vi "Day 5 (Part One).vi"() -> ()   [LabVIEW 2021]
panel:
  out "Result":string
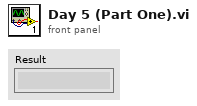
[diagram p1: front panel]
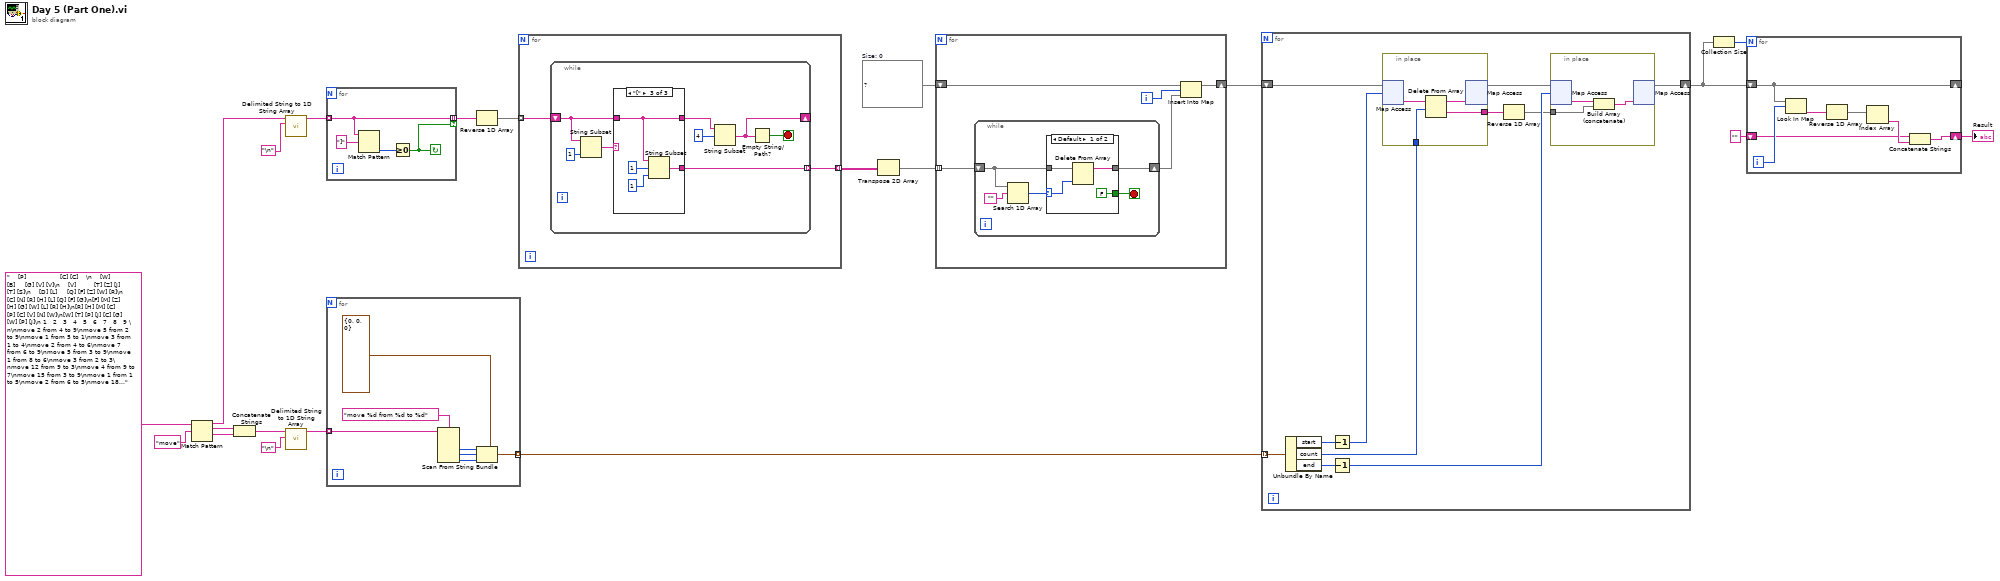
[diagram p0: block diagram]
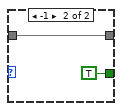
[diagram p2: hidden frame]
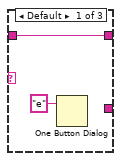
[diagram p3: hidden frame]
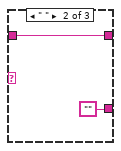
[diagram p4: hidden frame]
diagram:
  w7 = map{i32, string[]} {}  # Size: 0
  n1 = Match Pattern(string="    [P]                 [C] [C]    \n    [W]         [B]     [G] [V] [V]\n    [V]         [T] [Z] [J] [T] [S]\n    [D] [L]     [Q] [F] [Z] [W] [R]\n    [C] [N] [R] [H] [L] [Q] [F] [G]\n[F] [M] [Z] [H] [G] [W] [L] [R] [H]\n[R] [H] [M] [C] [P] [C] [V] [N] [W]\n[W] [T] [P] [J] [C] [G] [W] [P] [J]\n 1   2   3   4   5   6   7   8   9 \n\nmove 2 from 4 to 9\nmove 5 from 2 to 9\nmove 1 from 5 to 1\nmove 3 from 1 to 4\nmove 2 from 4 to 6\nmove 7 from 6 to 9\nmove 5 from 3 to 9\nmove 1 from 8 to 6\nmove 3 from 2 to 3\nmove 12 from 9 to 3\nmove 4 from 9 to 7\nmove 15 from 3 to 9\nmove 1 from 1 to 5\nmove 2 from 6 to 5\nmove 18 from 9 to 1\nmove 6 from 8 to 1\nmove 1 from 8 to 7\nmove 5 from 7 to 2\nmove 6 from 1 to 2\nmove 7 from 9 to 6\nmove 6 from 1 to 3\nmove 5 from 3 to 9\nmove 3 from 9 to 1\nmove 1 from 7 to 9\nmove 4 from 2 to 1\nmove 5 from 6 to 3\nmove 1 from 3 to 4\nmove 1 from 5 to 9\nmove 2 from 9 to 6\nmove 5 from 5 to 9\nmove 10 from 1 to 8\nmove 4 from 3 to 8\nmove 3 from 4 to 9\nmove 4 from 6 to 9\nmove 14 from 8 to 6\nmove 1 from 3 to 8\nmove 14 from 9 to 4\nmove 6 from 1 to 6\nmove 1 from 8 to 2\nmove 3 from 5 to 8\nmove 1 from 8 to 9\nmove 1 from 8 to 1\nmove 5 from 4 to 9\nmove 1 from 8 to 4\nmove 3 from 9 to 4\nmove 3 from 7 to 5\nmove 7 from 6 to 3\nmove 7 from 4 to 1\nmove 3 from 9 to 1\nmove 7 from 2 to 3\nmove 1 from 4 to 8\nmove 8 from 6 to 2\nmove 2 from 7 to 4\nmove 1 from 7 to 4\nmove 1 from 7 to 9\nmove 1 from 5 to 9\nmove 1 from 9 to 4\nmove 1 from 4 to 2\nmove 8 from 4 to 9\nmove 1 from 4 to 2\nmove 5 from 9 to 4\nmove 2 from 6 to 9\nmove 1 from 6 to 9\nmove 1 from 8 to 1\nmove 13 from 3 to 2\nmove 1 from 3 to 9\nmove 2 from 6 to 8\nmove 1 from 8 to 1\nmove 14 from 1 to 7\nmove 4 from 2 to 1\nmove 2 from 9 to 5\nmove 3 from 9 to 7\nmove 1 from 8 to 2\nmove 4 from 1 to 5\nmove 1 from 4 to 7\nmove 3 from 9 to 1\nmove 7 from 7 to 4\nmove 14 from 2 to 8\nmove 3 from 1 to 7\nmove 3 from 5 to 4\nmove 2 from 1 to 9\nmove 11 from 8 to 9\nmove 3 from 7 to 8\nmove 3 from 8 to 6\nmove 6 from 4 to 3\nmove 2 from 6 to 8\nmove 8 from 4 to 3\nmove 3 from 8 to 7\nmove 2 from 8 to 2\nmove 2 from 3 to 9\nmove 1 from 6 to 8\nmove 5 from 2 to 7\nmove 10 from 9 to 7\nmove 1 from 8 to 5\nmove 3 from 5 to 2\nmove 6 from 7 to 5\nmove 19 from 7 to 3\nmove 9 from 5 to 9\nmove 6 from 2 to 6\nmove 2 from 7 to 3\nmove 29 from 3 to 8\nmove 2 from 7 to 9\nmove 5 from 8 to 1\nmove 12 from 9 to 6\nmove 1 from 3 to 8\nmove 1 from 2 to 7\nmove 1 from 3 to 1\nmove 10 from 6 to 1\nmove 1 from 6 to 7\nmove 9 from 1 to 9\nmove 2 from 1 to 2\nmove 12 from 9 to 4\nmove 7 from 6 to 3\nmove 8 from 3 to 7\nmove 5 from 7 to 6\nmove 19 from 8 to 3\nmove 10 from 4 to 6\nmove 1 from 4 to 6\nmove 6 from 8 to 6\nmove 1 from 4 to 2\nmove 6 from 6 to 3\nmove 3 from 2 to 7\nmove 13 from 6 to 3\nmove 1 from 9 to 1\nmove 6 from 1 to 8\nmove 1 from 6 to 5\nmove 1 from 5 to 4\nmove 3 from 7 to 1\nmove 2 from 1 to 3\nmove 11 from 3 to 8\nmove 1 from 4 to 3\nmove 3 from 8 to 4\nmove 1 from 7 to 5\nmove 3 from 8 to 9\nmove 2 from 9 to 2\nmove 7 from 8 to 3\nmove 1 from 7 to 9\nmove 1 from 1 to 4\nmove 32 from 3 to 4\nmove 1 from 5 to 9\nmove 2 from 8 to 3\nmove 2 from 6 to 4\nmove 1 from 9 to 4\nmove 1 from 9 to 2\nmove 3 from 3 to 1\nmove 1 from 8 to 6\nmove 1 from 6 to 2\nmove 1 from 9 to 3\nmove 1 from 1 to 7\nmove 1 from 8 to 7\nmove 2 from 3 to 8\nmove 1 from 8 to 4\nmove 1 from 1 to 2\nmove 2 from 4 to 8\nmove 1 from 1 to 8\nmove 26 from 4 to 6\nmove 3 from 8 to 5\nmove 3 from 7 to 6\nmove 7 from 6 to 3\nmove 18 from 6 to 8\nmove 16 from 8 to 9\nmove 1 from 5 to 1\nmove 2 from 8 to 3\nmove 3 from 9 to 8\nmove 3 from 6 to 4\nmove 2 from 5 to 4\nmove 1 from 6 to 4\nmove 2 from 7 to 2\nmove 2 from 3 to 9\nmove 4 from 8 to 3\nmove 1 from 1 to 2\nmove 6 from 9 to 7\nmove 2 from 2 to 5\nmove 12 from 3 to 1\nmove 9 from 9 to 2\nmove 10 from 1 to 3\nmove 2 from 5 to 9\nmove 8 from 4 to 7\nmove 13 from 7 to 6\nmove 6 from 6 to 5\nmove 4 from 5 to 3\nmove 2 from 5 to 4\nmove 8 from 4 to 3\nmove 1 from 7 to 2\nmove 15 from 2 to 7\nmove 8 from 3 to 7\nmove 1 from 1 to 6\nmove 7 from 7 to 1\nmove 5 from 1 to 6\nmove 7 from 3 to 2\nmove 3 from 1 to 6\nmove 12 from 7 to 9\nmove 12 from 9 to 8\nmove 1 from 7 to 1\nmove 2 from 9 to 5\nmove 1 from 1 to 9\nmove 4 from 4 to 2\nmove 4 from 8 to 4\nmove 2 from 7 to 2\nmove 4 from 6 to 5\nmove 4 from 8 to 9\nmove 1 from 8 to 4\nmove 5 from 5 to 3\nmove 5 from 2 to 4\nmove 5 from 9 to 5\nmove 1 from 3 to 6\nmove 1 from 7 to 8\nmove 12 from 3 to 9\nmove 4 from 2 to 6\nmove 7 from 4 to 9\nmove 13 from 6 to 4\nmove 3 from 6 to 9\nmove 4 from 4 to 2\nmove 1 from 3 to 4\nmove 21 from 9 to 7\nmove 4 from 2 to 1\nmove 3 from 5 to 4\nmove 8 from 7 to 6\nmove 2 from 7 to 2\nmove 11 from 4 to 2\nmove 1 from 9 to 7\nmove 1 from 5 to 7\nmove 1 from 1 to 8\nmove 5 from 2 to 5\nmove 1 from 3 to 5\nmove 2 from 4 to 9\nmove 3 from 4 to 8\nmove 3 from 1 to 8\nmove 1 from 9 to 6\nmove 8 from 7 to 8\nmove 9 from 6 to 5\nmove 1 from 9 to 6\nmove 1 from 6 to 4\nmove 3 from 7 to 5\nmove 1 from 6 to 9\nmove 12 from 5 to 1\nmove 2 from 5 to 8\nmove 1 from 9 to 6\nmove 2 from 7 to 6\nmove 9 from 1 to 8\nmove 1 from 6 to 9\nmove 1 from 9 to 2\nmove 1 from 4 to 2\nmove 2 from 6 to 7\nmove 5 from 8 to 3\nmove 2 from 7 to 4\nmove 16 from 8 to 5\nmove 2 from 3 to 8\nmove 7 from 5 to 1\nmove 3 from 3 to 8\nmove 7 from 5 to 7\nmove 4 from 5 to 2\nmove 6 from 7 to 9\nmove 2 from 9 to 6\nmove 2 from 9 to 2\nmove 1 from 6 to 8\nmove 12 from 2 to 6\nmove 2 from 9 to 6\nmove 1 from 5 to 2\nmove 3 from 5 to 4\nmove 9 from 2 to 6\nmove 6 from 8 to 3\nmove 1 from 7 to 5\nmove 1 from 6 to 7\nmove 1 from 7 to 8\nmove 1 from 5 to 8\nmove 5 from 1 to 2\nmove 3 from 4 to 5\nmove 4 from 6 to 8\nmove 5 from 2 to 9\nmove 5 from 8 to 4\nmove 1 from 1 to 4\nmove 9 from 8 to 4\nmove 1 from 2 to 3\nmove 3 from 6 to 8\nmove 4 from 9 to 2\nmove 2 from 6 to 4\nmove 2 from 3 to 1\nmove 4 from 4 to 7\nmove 6 from 4 to 5\nmove 10 from 6 to 8\nmove 4 from 1 to 9\nmove 4 from 7 to 5\nmove 3 from 3 to 9\nmove 6 from 9 to 8\nmove 2 from 2 to 9\nmove 8 from 4 to 3\nmove 2 from 2 to 7\nmove 1 from 4 to 9\nmove 6 from 3 to 8\nmove 2 from 7 to 8\nmove 6 from 5 to 9\nmove 5 from 5 to 6\nmove 2 from 5 to 9\nmove 7 from 9 to 5\nmove 2 from 1 to 9\nmove 6 from 5 to 8\nmove 1 from 5 to 1\nmove 2 from 3 to 6\nmove 1 from 3 to 6\nmove 4 from 9 to 5\nmove 1 from 3 to 4\nmove 1 from 1 to 2\nmove 1 from 2 to 1\nmove 1 from 6 to 8\nmove 14 from 8 to 5\nmove 6 from 5 to 1\nmove 16 from 8 to 3\nmove 2 from 8 to 2\nmove 10 from 6 to 7\nmove 1 from 6 to 9\nmove 2 from 2 to 9\nmove 2 from 7 to 3\nmove 1 from 8 to 5\nmove 3 from 9 to 1\nmove 4 from 9 to 5\nmove 9 from 3 to 8\nmove 2 from 3 to 6\nmove 5 from 3 to 8\nmove 1 from 4 to 2\nmove 12 from 8 to 4\nmove 1 from 8 to 9\nmove 4 from 5 to 9\nmove 7 from 7 to 1\nmove 10 from 5 to 2\nmove 2 from 5 to 2\nmove 1 from 6 to 5\nmove 2 from 5 to 2\nmove 5 from 2 to 6\nmove 4 from 9 to 6\nmove 6 from 4 to 9\nmove 2 from 3 to 4\nmove 6 from 4 to 7\nmove 6 from 7 to 5\nmove 10 from 1 to 5\nmove 4 from 1 to 2\nmove 4 from 6 to 3\nmove 6 from 9 to 7\nmove 2 from 4 to 9\nmove 7 from 7 to 6\nmove 1 from 9 to 7\nmove 2 from 9 to 8\nmove 2 from 8 to 2\nmove 1 from 2 to 5\nmove 3 from 8 to 4\nmove 4 from 2 to 7\nmove 3 from 4 to 7\nmove 2 from 3 to 5\nmove 2 from 3 to 2\nmove 18 from 5 to 3\nmove 6 from 3 to 1\nmove 8 from 3 to 1\nmove 8 from 7 to 9\nmove 9 from 2 to 5\nmove 3 from 2 to 3\nmove 7 from 3 to 7\nmove 3 from 6 to 4\nmove 1 from 7 to 1\nmove 7 from 6 to 7\nmove 1 from 2 to 9\nmove 1 from 4 to 2\nmove 13 from 7 to 2\nmove 10 from 5 to 3\nmove 1 from 2 to 9\nmove 7 from 1 to 5\nmove 8 from 9 to 5\nmove 1 from 9 to 5\nmove 1 from 9 to 8\nmove 1 from 8 to 2\nmove 8 from 5 to 3\nmove 18 from 3 to 5\nmove 2 from 4 to 1\nmove 3 from 2 to 5\nmove 27 from 5 to 1\nmove 17 from 1 to 5\nmove 2 from 2 to 3\nmove 1 from 6 to 5\nmove 2 from 2 to 5\nmove 1 from 6 to 4\nmove 1 from 6 to 9\nmove 2 from 3 to 5\nmove 17 from 5 to 6\nmove 1 from 9 to 3\nmove 6 from 2 to 4\nmove 1 from 3 to 2\nmove 3 from 4 to 9\nmove 1 from 2 to 9\nmove 1 from 4 to 7\nmove 3 from 5 to 2\nmove 2 from 5 to 1\nmove 1 from 5 to 2\nmove 1 from 7 to 3\nmove 18 from 1 to 4\nmove 1 from 3 to 1\nmove 5 from 4 to 2\nmove 1 from 5 to 1\nmove 9 from 2 to 7\nmove 1 from 4 to 5\nmove 1 from 2 to 9\nmove 8 from 6 to 2\nmove 13 from 4 to 2\nmove 2 from 4 to 9\nmove 1 from 5 to 2\nmove 1 from 6 to 8\nmove 6 from 7 to 5\nmove 1 from 8 to 4\nmove 1 from 7 to 6\nmove 1 from 6 to 1\nmove 7 from 6 to 5\nmove 1 from 7 to 9\nmove 6 from 9 to 3\nmove 2 from 9 to 7\nmove 2 from 5 to 7\nmove 4 from 7 to 8\nmove 4 from 5 to 4\nmove 1 from 6 to 7\nmove 3 from 3 to 8\nmove 6 from 5 to 9\nmove 2 from 3 to 5\nmove 4 from 4 to 7\nmove 1 from 3 to 1\nmove 2 from 2 to 3\nmove 6 from 9 to 6\nmove 1 from 7 to 1\nmove 19 from 2 to 4\nmove 2 from 5 to 6\nmove 2 from 8 to 9\nmove 2 from 1 to 2\nmove 2 from 2 to 5\nmove 2 from 4 to 3\nmove 4 from 6 to 2\nmove 1 from 7 to 8\nmove 6 from 1 to 8\nmove 3 from 5 to 1\nmove 5 from 2 to 5\nmove 1 from 6 to 7\nmove 9 from 8 to 1\nmove 2 from 3 to 6\nmove 4 from 6 to 5\nmove 1 from 6 to 2\nmove 9 from 5 to 2\nmove 3 from 4 to 6\nmove 12 from 4 to 6\nmove 1 from 9 to 4\nmove 1 from 3 to 1\nmove 3 from 4 to 8\nmove 1 from 3 to 6\nmove 6 from 6 to 2\nmove 1 from 4 to 5\nmove 3 from 6 to 2\nmove 4 from 1 to 5\nmove 1 from 5 to 1\nmove 2 from 8 to 9\nmove 7 from 6 to 3\nmove 1 from 3 to 1\nmove 1 from 8 to 1\nmove 3 from 8 to 9\nmove 4 from 3 to 5\nmove 3 from 7 to 3\nmove 5 from 3 to 7\nmove 1 from 9 to 1\nmove 4 from 9 to 2\nmove 15 from 2 to 7\nmove 14 from 1 to 7\nmove 5 from 5 to 1\nmove 9 from 7 to 2\nmove 1 from 9 to 6\nmove 1 from 7 to 4\nmove 1 from 4 to 6\nmove 2 from 6 to 2\nmove 9 from 2 to 5\nmove 4 from 2 to 4\nmove 4 from 7 to 5\nmove 6 from 5 to 9\nmove 7 from 1 to 8\nmove 6 from 2 to 8\nmove 1 from 1 to 2\nmove 3 from 9 to 5\nmove 18 from 7 to 8\nmove 2 from 4 to 6\nmove 2 from 4 to 6\nmove 3 from 7 to 6\nmove 3 from 5 to 3\nmove 1 from 2 to 6\nmove 5 from 6 to 8\nmove 29 from 8 to 1\nmove 2 from 3 to 5\nmove 25 from 1 to 6\nmove 2 from 9 to 5\nmove 1 from 7 to 8\nmove 6 from 8 to 2\nmove 1 from 9 to 1\nmove 15 from 6 to 8\nmove 1 from 3 to 8\nmove 14 from 8 to 7\nmove 5 from 1 to 3\nmove 1 from 6 to 2\nmove 2 from 5 to 7\nmove 10 from 6 to 2\nmove 4 from 5 to 7\nmove 6 from 5 to 1\nmove 2 from 1 to 4\nmove 19 from 7 to 9", regular expression="move") -> (before substring=w13:string, match substring=w19:string, after substring=w18:string)  [unwired: 1 in, 1 out]
  n2 = Concatenate Strings(w19, w18) -> (w17:string)
  n3 = call <vilib>:"Delimited String to 1D String Array.vi"("delimiter"="\n", "delimited string"=w13) -> ("string array"=w12:string[])  [unwired: 9 in]
  n4 = call <vilib>:"Delimited String to 1D String Array.vi"("delimiter"="\n", "delimited string"=w17) -> ("string array"=w15:string[])  [unwired: 9 in]
  n5 = for {
    tunnel: w12 -> [w23] mode=indexing
    tunnel: [w23] -> w11 mode=indexing if=w22
    stop <- w22 continue-if-true
    n6 = Match Pattern(string=w23, regular expression="]") -> (offset past match=w24:i32)  [unwired: 1 in, 3 out]
    n7 = Greater Or Equal To 0?(x=w24) -> (x >= 0?=w22:bool)
  }
  n8 = for {
    tunnel: w15 -> [w32] mode=indexing
    tunnel: [w26] -> w9 mode=indexing
    n9 = Scan From String(format string="move %d from %d to %d", input string=w32) -> (output 1=w29:i32, output 2=w28:i32, output 3=w27:i32)  [unwired: 5 in, 3 out]
    n10 = Bundle(cluster=cluster{"count":i32, "start":i32, "end":i32} {"count"=0, "start"=0, "end"=0}, "count"=w29, "start"=w28, "end"=w27) -> (w26:cluster{"count":i32, "start":i32, "end":i32})
  }
  n11 = Reverse 1D Array(array=w11) -> (reversed array=w10:string[])
  n12 = for {
    tunnel: w10 -> [w34] mode=indexing
    tunnel: [w33] -> w8 mode=indexing
    n13 = while {
      shift-right: [w35] -> _
      shift-left: w34 -> [w40]
      tunnel: [w39] -> w33 mode=indexing
      stop <- w38 stop-if-true
      n14 = String Subset(string=w40, length (rest)=1 ("length (rest)")) -> (substring=w41:string)  [unwired: 1 in]
      n15 = case shown="\"[\"" w41 {
        tunnel: w40 -> [w43 w45 w47]
        tunnel: [_ "" ("String") w48] -> w39
        tunnel: [w43 w45 w47] -> w36
        frame Default {
          n16 = One Button Dialog(message="e") -> ()  [unwired: 1 in, 1 out]
        }
        frame " " {
        }
        frame "[" {
          n17 = String Subset(string=w47, offset (0)=1, length (rest)=1 ("length (rest)")) -> (substring=w48:string)
        }
      }
      n18 = String Subset(string=w36, offset (0)=4) -> (substring=w35:string)  [unwired: 1 in]
      n19 = Empty String/Path?(string/path=w35) -> (empty?=w38:bool)
    }
  }
  n20 = Transpose 2D Array(2D array=w8) -> (transposed array=w6:string[][])
  n21 = for {
    shift-right: [w51] -> w5
    shift-left: w7 -> [w54]
    tunnel: w6 -> [w55] mode=indexing
    i -> [w52]
    n22 = while {
      shift-right: [w57] -> w53
      shift-left: w55 -> [w58]
      stop <- w56 stop-if-true
      n23 = Search 1D Array(1D array=w58, element="") -> (index of element=w59:i32)  [unwired: 1 in]
      n24 = case shown="Default" w59 {
        selector: w59 -> [w63 _]
        tunnel: w58 -> [w64 w66]
        tunnel: [w62 w66] -> w57
        tunnel: [FALSE TRUE] -> w56
        frame Default {
          n25 = Delete From Array(array=w64, index=w63) -> (array with subset deleted=w62:string[])  [unwired: 1 in, 1 out]
        }
        frame -1 {
        }
      }
    }
    n26 = Insert Into Map(map in=w54, key=w52, value=w53) -> (map out=w51:map{i32, string[]})  [unwired: 2 out]
  }
  n27 = for {
    tunnel: w9 -> [w75] mode=indexing
    shift-right: [w68] -> w4
    shift-left: w5 -> [w74]
    n28 = Unbundle By Name(w75) -> ("start"=w76:i32, "count"=w72:i32, "end"=w77:i32)
    n29 = Decrement(x=w76) -> (x-1=w73:i32)
    n30 = Decrement(x=w77) -> (x-1=w70:i32)
    n31 = in-place {
      in-place-border: w72 -> [w83]
      in-place-border: [w81] -> w69
      n32 = in-place-map #1(w74, w73) -> (w84:string[])  [unwired: 1 in, 1 out]
      n33 = Delete From Array(array=w84, length=w83) -> (deleted portion=w81:string[], array with subset deleted=w82:string[])  [unwired: 1 in]
      n34 = in-place-map #1(w82) -> (w71:map{i32, string[]})  [unwired: 1 in, 2 out]
    }
    n35 = Reverse 1D Array(array=w69) -> (reversed array=w67:string[])
    n36 = in-place {
      in-place-border: w67 -> [w79]
      n37 = in-place-map #2(w71, w70) -> (w80:string[])  [unwired: 1 in, 1 out]
      n38 = Build Array (concatenate)(w80, w79) -> (w78:string[])
      n39 = in-place-map #2(w78) -> (w68:map{i32, string[]})  [unwired: 1 in, 2 out]
    }
  }
  n40 = Collection Size(1:w4) -> (0:w3:i32)
  n41 = for {
    N: w3 -> [_]
    shift-right: [w88] -> _
    shift-left: w4 -> [w88]
    shift-right: [w86] -> w2
    shift-left: "" -> [w85]
    i -> [w91]
    n42 = Look In Map(map=w88, key=w91) -> (value=w90:string[])  [unwired: 1 in, 1 out]
    n43 = Reverse 1D Array(array=w90) -> (reversed array=w89:string[])
    n44 = Index Array(array=w89) -> (element=w87:string)  [unwired: 1 in]
    n45 = Concatenate Strings(w85, w87) -> (w86:string)
  }
  "Result" <- w2
